vi "SwerveDrivePoseEst_BiConsum_VisionCorrect.vi"(9 "Y":T2, 10 "U":T2, 11 "ExtraPassedData":variant) -> (0 "Error":bool, 3 "ExtraReturnedData":variant)   [LabVIEW 2019, in "Trajectory_Library.lvlib"]
doc: "Function used by LatencyCompensator_ApplyPastGlobalMeasurement\n\nThis is a work in progress!!"
uses:
  Trajectory_Library.lvlib
  <vilib>/Analysis/Matrix/Datatypes/RealMatrix.ctl
  UNSCENTED_KALMAN_FILTER.ctl
  MERWE_SCALED_SIGMA_PTS.ctl
  BiFun_Matrix_FUNC_TYPE.ctl
  AngleStats_AngleMean_BiFunc.vi
  AngleStats_AngleResidual_BiFunc.vi
  AngleStats_AngleAdd_BiFunc.vi
  SwerveDrivePoseEst_BiFunc_F.vi
  <vilib>/Analysis/Matrix/NI_Matrix.lvlib
panel:
  in  "Cluster":T5
  # "State Estimate <Statess,1>"
  # "<States, States>"
  # "<States, ?>"
  # "<Statess,  States>"
  # "<Outputs, Outputs>"
  # "<?, 1>"
  # "<?, 1>"
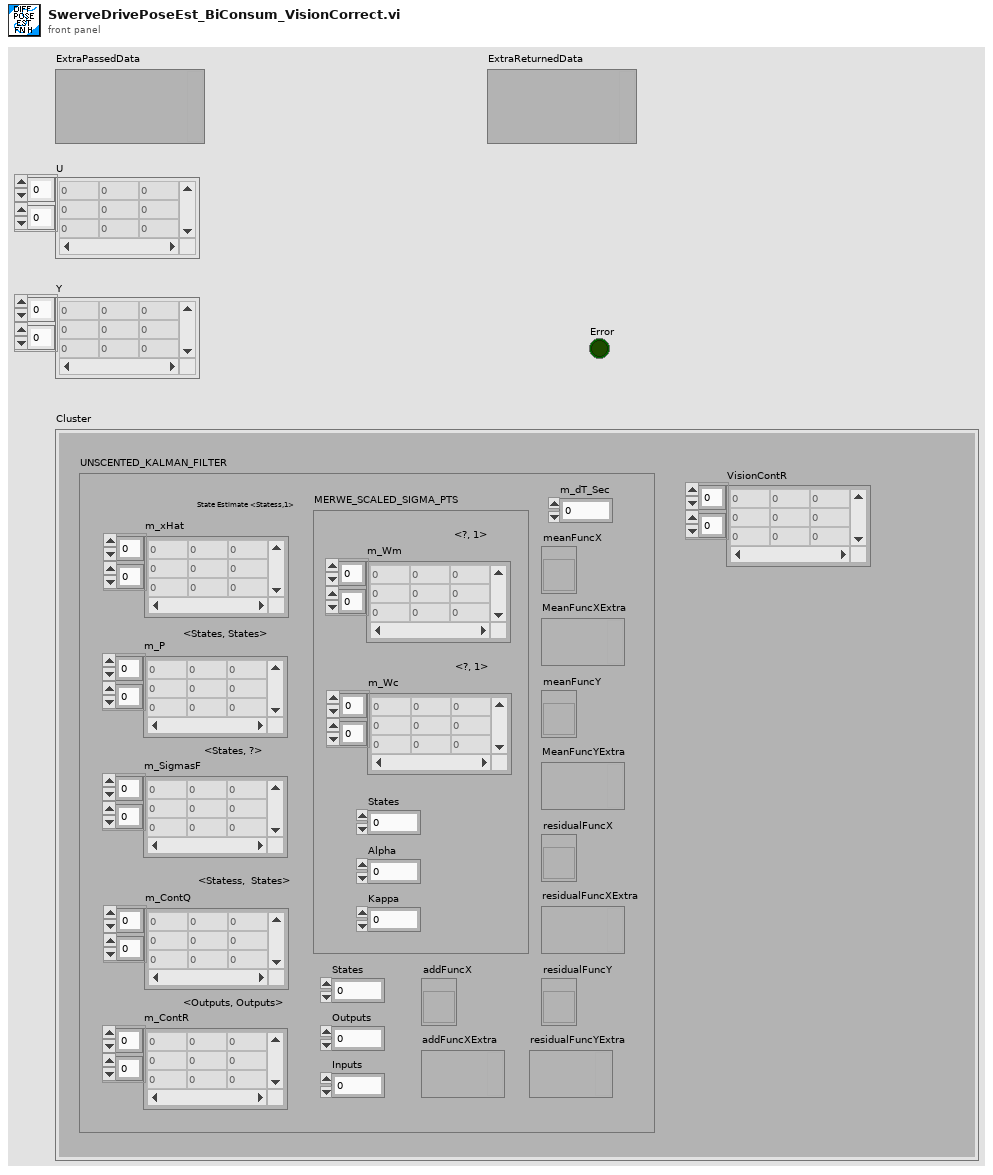
[diagram p1: front panel]
types:
  T1 = typedef "Trajectory_Library.lvlib/UNSCENTED_KALMAN_FILTER.ctl" = cluster{"m_P":T2, "m_xHat":T2, "States":i32, "Outputs":i32, "m_ContR":T2, "m_ContQ":T2, "m_SigmasF":T2, "m_dT_Sec":dbl, "MERWE_SCALED_SIGMA_PTS":T3, "meanFuncX":T4, "meanFuncY":T4, "residualFuncX":T4, "residualFuncY":T4, "addFuncX":T4, "addFuncXExtra":variant, "residualFuncYExtra":variant, "residualFuncXExtra":variant, "MeanFuncYExtra":variant, "MeanFuncXExtra":variant, "Inputs":i32}
  T2 = typedef "NI_Matrix.lvlib/RealMatrix.ctl" = dbl[][]
  T3 = typedef "Trajectory_Library.lvlib/MERWE_SCALED_SIGMA_PTS.ctl" = cluster{"m_Wm":T2, "States":i32, "Alpha":dbl, "m_Wc":T2, "Kappa":i32}
  T4 = typedef "Trajectory_Library.lvlib/BiFun_Matrix_FUNC_TYPE.ctl" = refnum<vi>
  T5 = cluster{"UNSCENTED_KALMAN_FILTER":T1, "VisionContR":T2}
  T6 = typedef "Trajectory_Library.lvlib/UNSCENTED_KALMAN_CORRECT_FUNC_GROUP.ctl" = cluster{"H_Func":T4, "meanFuncY":T4, "residualFuncY":T4, "residualFuncX":T4, "addFuncX":T4, "H_FuncExtra":variant, "MeanFuncYExtra":variant, "residualFuncYExtra":variant, "residualFuncXExtra":variant, "addFuncXExtra":variant}
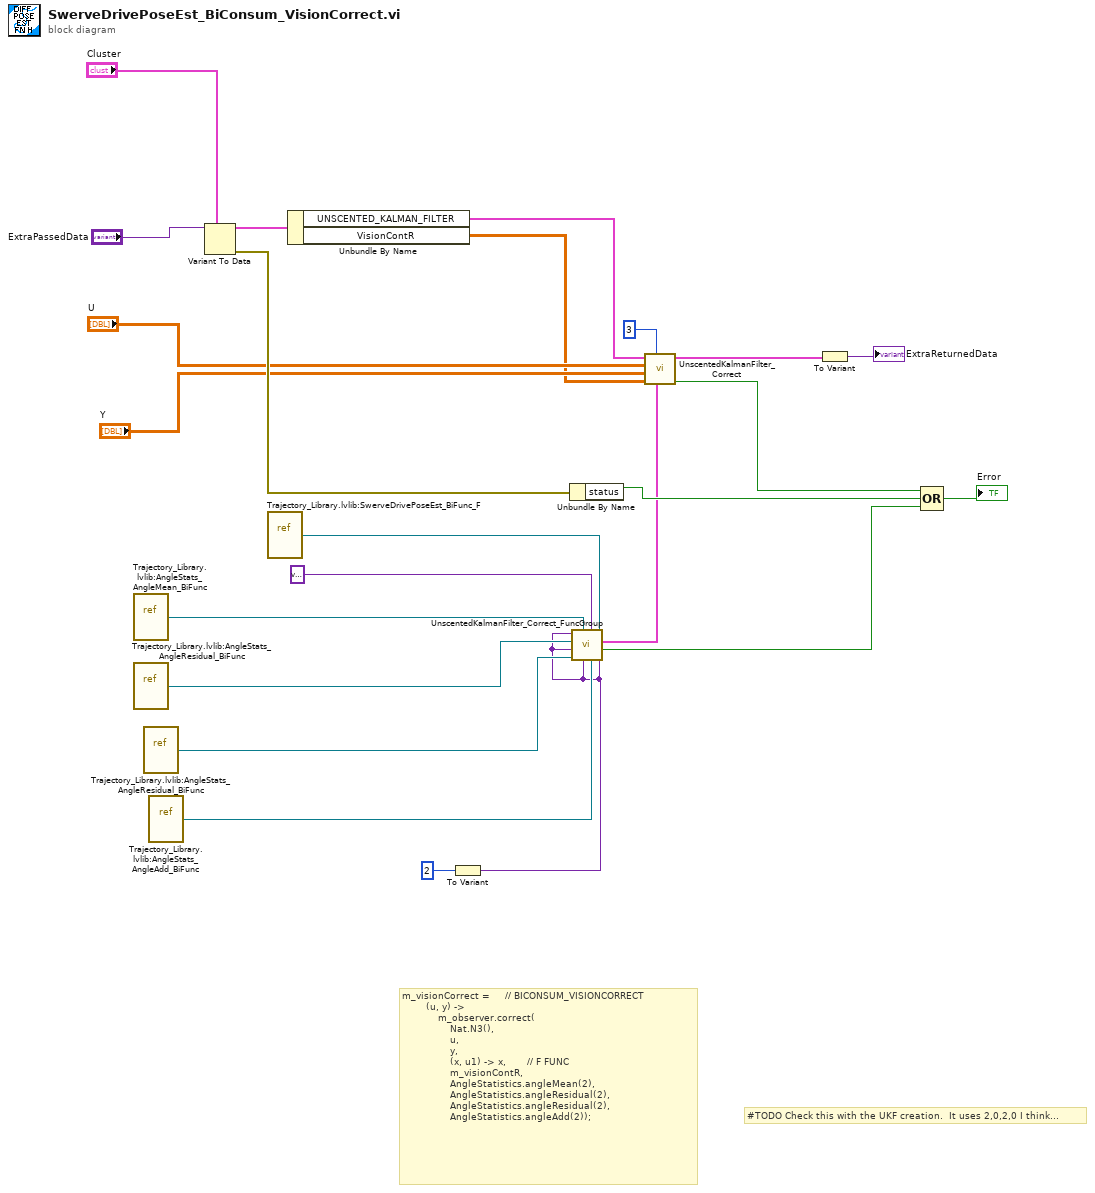
[diagram p0: block diagram]
diagram:
  # "#TODO Check this with the UKF creation.  It uses 2,0,2,0 I think..."
  # "m_visionCorrect =\t\t\t\t\t// BICONSUM_VISIONCORRECT \n        (u, y) ->\n            m_observer.correct(\n                Nat.N3(),\n                u,\n                y,\n                (x, u1) -> x,       // F FUNC\n                m_visionContR,\n                AngleStatistics.angleMean(2),\n                AngleStatistics.angleResidual(2),\n                AngleStatistics.angleResidual(2),\n                AngleStatistics.angleAdd(2));"
  n1 = vi-ref "Trajectory_Library.lvlib:AngleStats_AngleMean_BiFunc.vi"() -> (w5:refnum<vi>)
  n2 = vi-ref "Trajectory_Library.lvlib:AngleStats_AngleResidual_BiFunc.vi"() -> (w6:refnum<vi>)
  n3 = vi-ref "Trajectory_Library.lvlib:AngleStats_AngleResidual_BiFunc.vi"() -> (w7:refnum<vi>)
  n4 = vi-ref "Trajectory_Library.lvlib:AngleStats_AngleAdd_BiFunc.vi"() -> (w8:refnum<vi>)
  n5 = Variant To Data(type="Cluster", Variant="ExtraPassedData") -> (data=w22:T5, error out=w18:errorcluster)  [unwired: 1 in]
  n6 = vi-ref "Trajectory_Library.lvlib:SwerveDrivePoseEst_BiFunc_F.vi"() -> (w1:refnum<vi>)
  n7 = Unbundle By Name(w22) -> ("UNSCENTED_KALMAN_FILTER"=w20:T1, "VisionContR"=w12:T2)
  n8 = To Variant(anything=2) -> (Variant=w2:variant)
  n9 = Unbundle By Name(w18) -> ("status"=w17:bool)
  n10 = call "UnscentedKalmanFilter_Correct_FuncGroup.vi"("addFuncXExtra"=w2, "H_Func"=w1, "AddFuncX"=w8, "H_FuncExtra"=variant ("F_Func_ExtraData"), "residualFuncXExtra"=w2, "MeanFuncY"=w5, "ResidualFuncX"=w7, "residualFuncYExtra"=w2, "ResidualFuncY"=w6, "MeanFuncYExtra"=w2) -> ("Error"=w4:bool, "UNSCENTED_KALMAN_CORRECT_FUNC_GROUP"=w13:T6)
  n11 = call "UnscentedKalmanFilter_Correct.vi"("UNSCENTED_KALMAN_CORRECT_FUNC_GROUP"=w13, "Rows"=3, "R"=w12, "Y"="Y", "U"="U", "in UnscentedKalmanFiilter"=w20) -> ("Error"=w16:bool, "out UnscentedKalmanFiilter"=w9:T1)  [unwired: 4 in]
  n12 = To Variant(anything=w9) -> (Variant=→"ExtraReturnedData":variant)
  n13 = Compound Arithmetic op=OR(w16, w17, w4) -> (→"Error":bool)
